vi "Read HistoryData.vi"(8 "error in":errorcluster caption="错误输入（无错误）", 10 "Channel Tag[]":string[](array[string])) -> (0 "error out":errorcluster caption="错误输出", 2 "Waveform":waveform(dbl)[](array[waveform]))   [LabVIEW 2016]
uses:
  DataReview/Controls/Read Condition.ctl
  GlobleVariables/GlobleVariables.vi
  GlobleVariables/Ctrl_Sample Configure.ctl
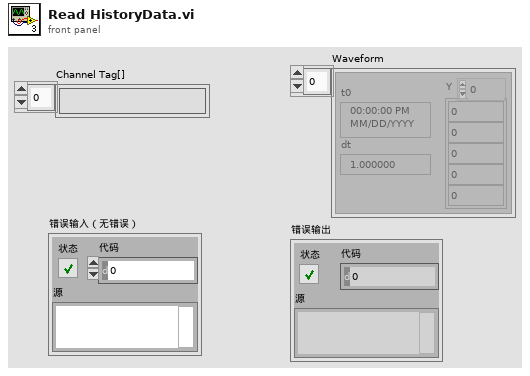
[diagram p1: front panel]
types:
  T1 = typedef "Ctrl_Sample Configure.ctl" = enum16{"Read", "Set"}
  T2 = typedef "Read Condition.ctl" = cluster{"Read Center Time":timestamp, "Read Start Time":timestamp, "Read End Time":timestamp, "Group Name":string, "Channel Names":string[]}
  T3 = typedef "ConfigureInfo.ctl" = cluster{"System":T4, "Signal[]":T5[], "Analyze Set":T6}
  T4 = typedef "System Config Information.ctl" = cluster{"测试名称":string, "存储文件夹路径":path, "存储时间间隔(min)":dbl, "采样率(HZ)":dbl, "非动态信号采样率(HZ)":dbl, "数据刷新频率(HZ)":dbl, "默认波形图个数":u8}
  T5 = typedef "Signal Information.ctl" = cluster{"Signal Type":string, "Channels Tag":string[], "Channels Name":string[], "Unit":string[], "Alarm Upper Limit":dbl[], "Alarm Lower Limit":dbl[], "Sensitivity":dbl[], "SampleRate":dbl[], "Sensor":string[], "FilterFreq":string[], "InputMode":string[], "AntiAliasingFilter":string[]}
  T6 = typedef "Analyze Set.ctl" = cluster{"FFT Set":T7, "Power Set":T8, "Shock Set":T9}
  T7 = typedef "FFT Set.ctl" = cluster{"F-W":enum16{"None", "Hanning", "Hamming", "Blackman-Harris", "Exact Blackman", "Blackman", "Flat Top", "4 Term B-Harris ", "7 Term B-Harris", "Low Sidelobe", "Force", "Exponential", "Blackman Nuttall", "Triangle", "Bartlett-Hanning", "Bohman", "Parzen", "Welch", "Kaiser", "Dolph-Chebyshev", "Gaussian"}, "F-L":dbl, "F-R":dbl}
  T8 = typedef "Power Set.ctl" = cluster{"P-W":enum16{"None", "Hanning", "Hamming", "Blackman-Harris", "Exact Blackman", "Blackman", "Flat Top", "4 Term B-Harris ", "7 Term B-Harris", "Low Sidelobe", "Force", "Exponential", "Blackman Nuttall", "Triangle", "Bartlett-Hanning", "Bohman", "Parzen", "Welch", "Kaiser", "Dolph-Chebyshev", "Gaussian"}, "P-L":dbl, "P-R":dbl}
  T9 = typedef "Shock Set.ctl" = cluster{"S-W":enum16{"None", "Hanning", "Hamming", "Blackman-Harris", "Exact Blackman", "Blackman", "Flat Top", "4 Term B-Harris ", "7 Term B-Harris", "Low Sidelobe", "Force", "Exponential", "Blackman Nuttall", "Triangle", "Bartlett-Hanning", "Bohman", "Parzen", "Welch", "Kaiser", "Dolph-Chebyshev", "Gaussian"}, "S-L":dbl, "S-R":dbl, "S-Z":dbl, "S-FFT":dbl}
  T10 = typedef "Folder Information.ctl" = cluster{"Folder Info":T11, "File Information":T12[], "Group Information":T13[]}
  T11 = typedef "TDMS File Info.ctl" = cluster{"Path":path, "Start Time":timestamp, "End Time":timestamp, "TdmsRef":refnum<k34>}
  T12 = typedef "File Information.ctl" = cluster{"File":T11, "Groups":T13[]}
  T13 = typedef "Group Information.ctl" = cluster{"Group Name":string, "Channel Names":string[], "Channel Units":string[], "dt":dbl, "Length":u64}
  T14 = typedef "File Read Parameters.ctl" = cluster{"File Parameters":T15[], "Read Condition":T2}
  T15 = typedef "Single File Read Parameter.ctl" = cluster{"File Read Information":T16, "File Information":T12}
  T16 = typedef "File Read Information.ctl" = cluster{"Zero?":bool, "Zero":i64, "Read?":bool, "Offset":i64, "Length":i64}
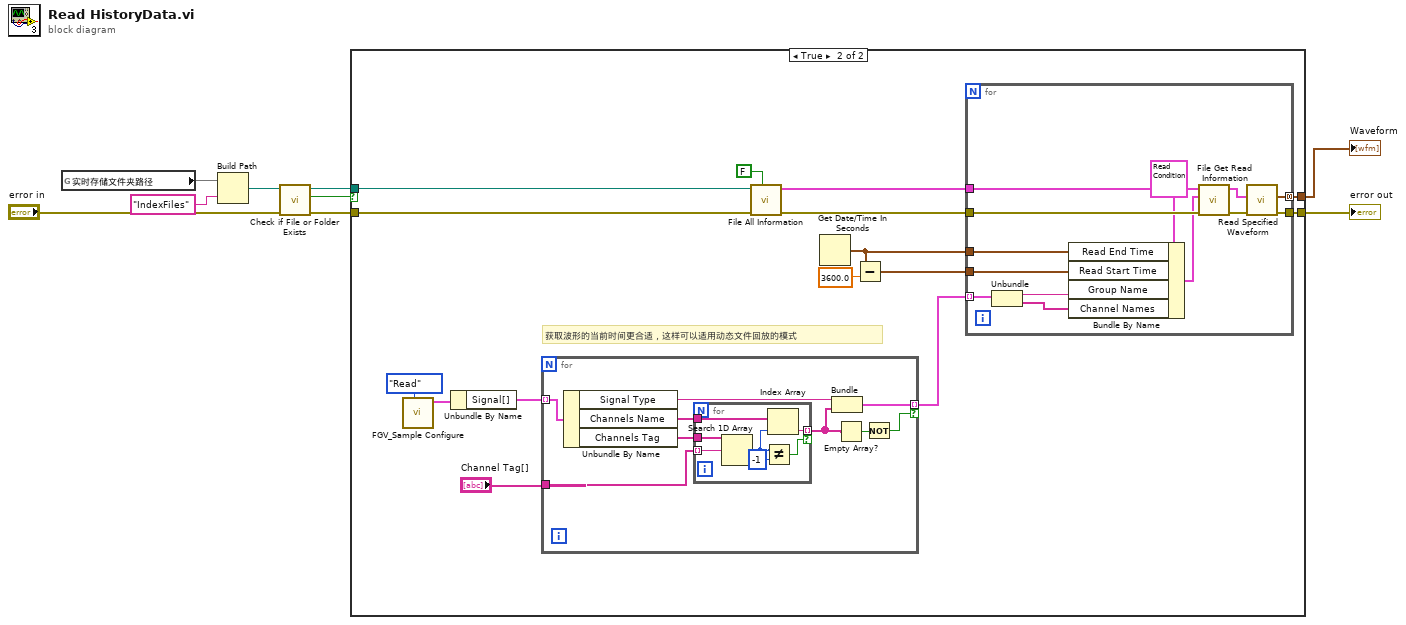
[diagram p0: block diagram]
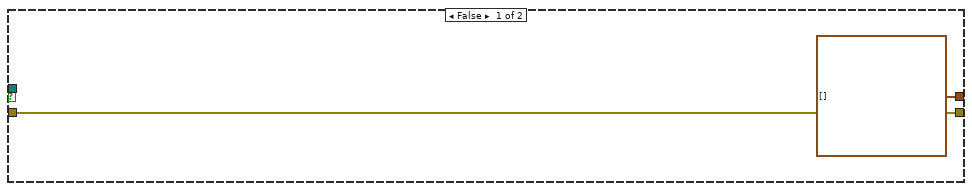
[diagram p2: hidden frame]
diagram:
  n1 = global read "GlobleVariables.vi" "实时存储文件夹路径"() -> (w9)
  n2 = Build Path(base path=w9, name or relative path="IndexFiles" ("名称或相对路径")) -> (appended path=w5:path)
  n3 = call <vilib>:"Check if File or Folder Exists.vi"("error in (no error)"="error in", "path"=w5) -> ("error out"=w2:errorcluster, "file or folder exists?"=w1:bool, "dup path"=w4:path)  [unwired: 7 in]
  n4 = case shown="True" w1 {
    tunnel: [waveform(dbl)[] [] ("Waveform") w24] -> w7
    tunnel: [w11 w23] -> w6
    tunnel: w4 -> [_ w14]
    tunnel: w2 -> [w11 w13]
    frame False {
    }
    frame True {
      # "获取波形的当前时间更合适，这样可以适用动态文件回放的模式"
      n5 = call "FGV_Sample Configure.vi"("Action"=Ctrl_Sample_Configure."Read") -> ("ConfigureInfo"=w20:T3)  [unwired: 9 in, 1 out]
      n6 = Unbundle By Name(w20) -> ("Signal[]"=w19:T5[])
      n7 = for {
        tunnel: "Channel Tag[]" -> [w48]
        tunnel: w19 -> [w47] mode=indexing
        tunnel: [w43] -> w18 mode=indexing if=w40
        n8 = Unbundle By Name(w47) -> ("Signal Type"=w44:string, "Channels Name"=w45:string[], "Channels Tag"=w46:string[])
        n9 = for {
          tunnel: w48 -> [w55] mode=indexing
          tunnel: w46 -> [w54]
          tunnel: w45 -> [w53]
          tunnel: [w52] -> w42 mode=indexing if=w49
          n10 = Search 1D Array(1D array=w54, element=w55) -> (index of element=w51:i32)  [unwired: 1 in]
          n11 = Not Equal?(x=w51, y=-1) -> (x != y?=w49:bool)
          n12 = Index Array(array=w53, index=w51) -> (element=w52:string)
        }
        n13 = Bundle("Signal Type"=w44, w42) -> (w43:cluster{"Signal Type":string, string[]})  [unwired: 1 in]
        n14 = Empty Array?(array=w42) -> (empty?=w41:bool)
        n15 = Not(x=w41) -> (.not. x?=w40:bool)
      }
      n16 = call "File All Information.vi"("Auto"=FALSE, "error in"=w13, "FoldPath"=w14) -> ("error out"=w26:errorcluster, "Folder Information"=w25:T10)  [unwired: 5 in, 2 out]
      n17 = Get Date/Time In Seconds() -> (seconds since 1Jan1904=w17:timestamp)
      n18 = Subtract(x=w17, y=3600.0) -> (x-y=w16:timestamp)
      n19 = for {
        tunnel: w26 -> [w37]
        tunnel: w25 -> [w36]
        tunnel: [w33] -> w24 mode=concatenating
        tunnel: [w32] -> w23
        tunnel: w18 -> [w31] mode=indexing
        tunnel: w17 -> [w28]
        tunnel: w16 -> [w27]
        n20 = Unbundle(w31) -> ("Signal Type"=w30:string, w29:string[])
        n21 = Bundle By Name(cluster=T2 {"Read Center Time"=timestamp(0 s since 1904-01-01), "Read Start Time"=timestamp(0 s since 1904-01-01), "Read End Time"=timestamp(0 s since 1904-01-01), "Group Name"="", "Channel Names"=[]} ("Read Condition"), "Read End Time"=w28, "Read Start Time"=w27, "Group Name"=w30, "Channel Names"=w29) -> (w34:T2)
        n22 = call "File Get Read Information.vi"("error in (no error)"=w37, "Read Condition"=w34, "Folder Information"=w36) -> ("error out"=w39:errorcluster, "Read Parameters"=w38:T14)  [unwired: 6 in, 1 out]
        n23 = call "Read Specified Waveform.vi"("error in"=w39, "Read Parameters"=w38) -> ("error out"=w32:errorcluster, "Waveform"=w33:waveform(sgl)[])  [unwired: 7 in, 1 out]
      }
    }
  }
  "Waveform" <- w7
  "error out" <- w6
